vi "Get Cursor Position.vi"(11 "Base Graph in":refnum<class "Base Graph.lvclass">) -> (2 "Cursor Position":T1, 3 "Base Graph out":refnum<class "Base Graph.lvclass">)   [LabVIEW 2023, in "Base Graph.lvclass"]
uses:
  Base Graph.lvclass
  <vilib>/Utility/miscctls.llb/LVPointDoubleTypeDef.ctl
  Base Graph.lvclass/Base Graph.ctl
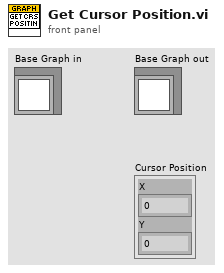
[diagram p1: front panel]
types:
  T1 = typedef "LVPointDoubleTypeDef.ctl" = cluster{"X":dbl, "Y":dbl}
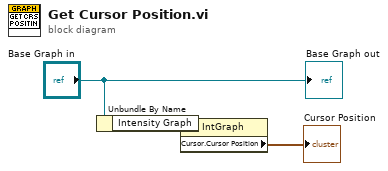
[diagram p0: block diagram]
diagram:
  n1 = Unbundle By Name("Base Graph in") -> ("Intensity Graph"=w2:refnum<vi>)
  n2 = property class="IntGraph"(reference=w2) -> ("Cursor.Cursor Position"=→"Cursor Position":T1)  [unwired: 1 in, 2 out]
  "Base Graph out" <- "Base Graph in"
